vi "Default Data.vi"(2 "Num Rows":i32, 3 "Pulseblaster in":refnum<class "Pulseblaster.lvclass">) -> (0 "Default Data":string[][](table), 1 "Pulseblaster out":refnum<class "Pulseblaster.lvclass">)   [LabVIEW 2013, in "Pulseblaster.lvclass"]
uses:
  Pulseblaster.lvclass
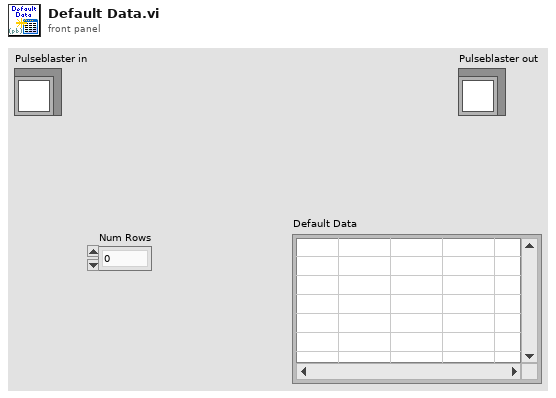
[diagram p1: front panel]
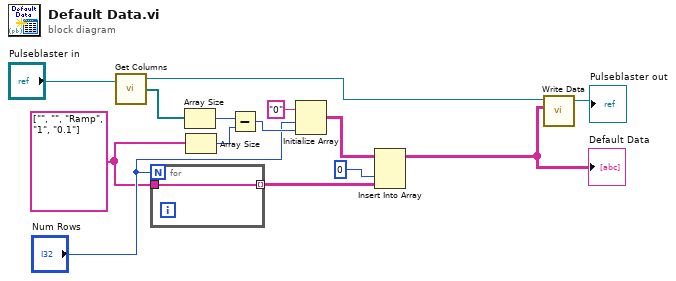
[diagram p0: block diagram]
diagram:
  w5 = string[] ["", "", "Ramp", "1", "0.1"]
  n1 = call-dynamic "Get Columns.vi"("Device in"="Pulseblaster in") -> ("Device out"=w10:refnum<class "Pulseblaster.lvclass">, "Columns"=w14:refnum<class "Column.lvclass">[])  [unwired: 1 in, 1 out]
  n2 = for {
    N: "Num Rows" -> [_]
    tunnel: w5 -> [w15]
    tunnel: [w15] -> w2 mode=indexing
  }
  n3 = Array Size(array=w14) -> (size(s)=w8:i32)
  n4 = Array Size(array=w5) -> (size(s)=w9:i32)
  n5 = Subtract(x=w8, y=w9) -> (x-y=w7:i32)
  n6 = Initialize Array("0", "Num Rows", w7) -> (w3:string[][])
  n7 = Insert Into Array(array=w3, index (col)=0 ("disabled index (col)"), new element=w2) -> (w4:string[][])  [unwired: 1 in]
  "Default Data" <- w4
  n8 = call-dynamic "Write Data.vi"("Data"=w4, "Device in"=w10) -> ("Device Out"=→"Pulseblaster out":refnum<class "Pulseblaster.lvclass">)  [unwired: 8 in, 1 out]
